vi "add_status.vi"(10 "string":string, 11 "Status Ref":refnum<vi>) -> ()   [LabVIEW 2020]
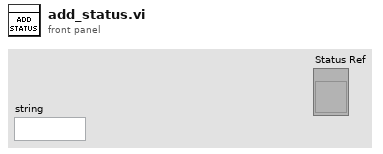
[diagram p1: front panel]
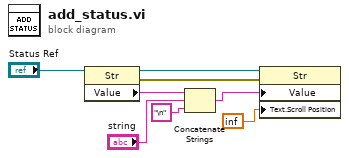
[diagram p0: block diagram]
diagram:
  n1 = property class="Str"(reference="Status Ref") -> (reference out=w4:refnum<vi>, error out=w5:errorcluster, "Value"=w6:string)  [unwired: 1 in]
  n2 = Concatenate Strings(w6, "string", "\n" ("string")) -> (w7:string)
  n3 = property class="Str"(reference=w4, error in=w5, "Value"=w7, "Text.Scroll Position"=inf) -> ()  [unwired: 2 out]
